vi "Run Test - Seconds to Time Stirngs (SubVI).vi"(11 "Seconds":sgl) -> (3 "Time Strings":string)   [LabVIEW 2019]
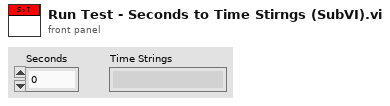
[diagram p1: front panel]
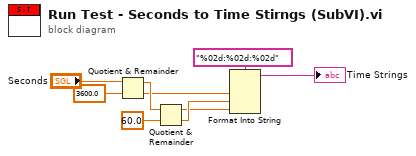
[diagram p0: block diagram]
diagram:
  n1 = Quotient & Remainder(x="Seconds", y=sgl 3600.0) -> (x-y*floor(x/y)=w8:sgl, floor(x/y)=w6:sgl)
  n2 = Quotient & Remainder(x=w8, y=sgl 60.0) -> (x-y*floor(x/y)=w4:sgl, floor(x/y)=w5:sgl)
  n3 = Format Into String(format string="%02d:%02d:%02d" ("Format String"), w6, w5, w4) -> (resulting string=→"Time Strings":string)  [unwired: 2 in, 1 out]
